vi "VSCode-dummy.vi"(11 "Enter your IP address":string="10.0.0.161") -> (0 "output cluster":errorcluster, 3 "standard output":string="Linux ev3dev 4.14.117-ev3dev-2.3.4-ev3 #1 PREEMPT Thu May 9 15:13:01 CDT 2019 armv5tejl\n             _____     _\n   _____   _|___ /  __| | _____   __\n  / _ \\ \\ / / |_ \\ / _` |/ _ \\ \\ / /\n |  __/\\ V / ___) | (_| |  __/\\ V /\n  \\___| \\_/ |____/ \\__,_|\\___| \\_/\n\nDebian stretch on LEGO MINDSTORMS EV3!\n")   [LabVIEW 2019]
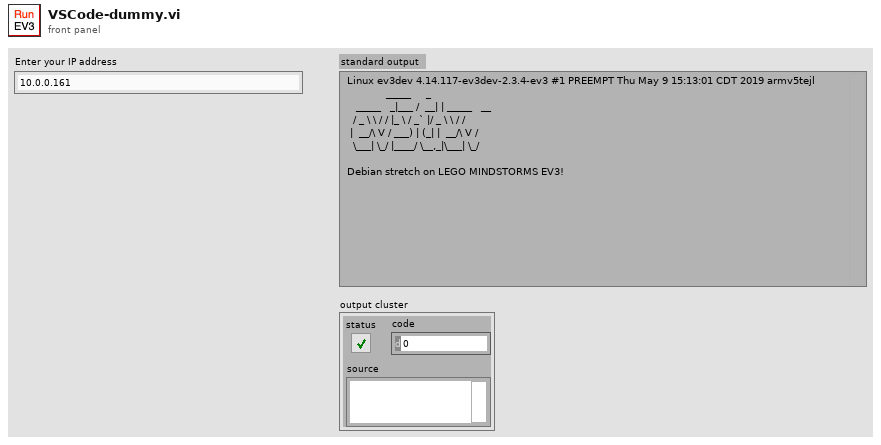
[diagram p1: front panel]
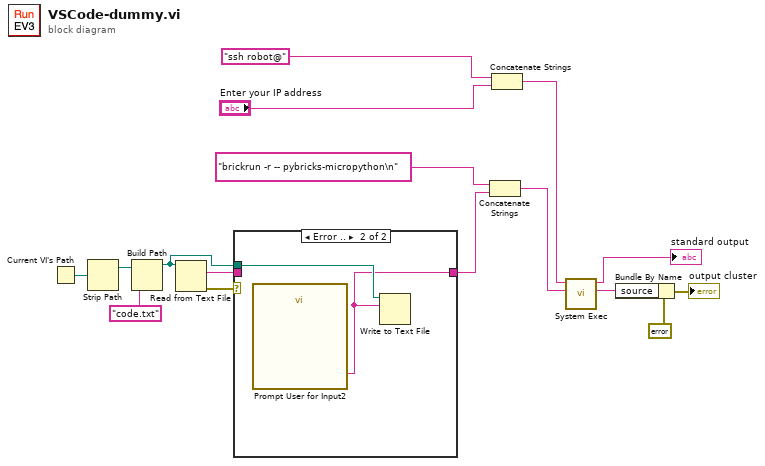
[diagram p0: block diagram]
diagram:
  n1 = Current VI's Path() -> (path=w15:path)
  n2 = Strip Path(path=w15) -> (stripped path=w14:path)  [unwired: 1 out]
  n3 = Build Path(base path=w14, name or relative path="code.txt") -> (appended path=w1:path)
  n4 = Read from Text File(file (use dialog)=w1) -> (text=w2:string, error out=w4:errorcluster)  [unwired: 3 in, 2 out]
  n5 = case shown="Error .." w4 {
    tunnel: w1 -> [_ w19]
    tunnel: [w17 w18] -> w3
    tunnel: w2 -> [w17 _]
    frame No Error {
    }
    frame Error {
      n6 = call "Prompt User for Input2"() -> ("code"=w18:string)  [unwired: 17 in, 2 out]
      n7 = Write to Text File(file (use dialog)=w19, text=w18) -> ()  [unwired: 2 in, 3 out]
    }
  }
  n8 = Concatenate Strings("brickrun -r -- pybricks-micropython\n" ("standard input"), w3) -> (w12:string)
  n9 = Concatenate Strings("ssh robot@" ("command line"), "Enter your IP address") -> (w11:string)
  n10 = call <vilib>:"System Exec.vi"("standard input"=w12, "command line"=w11) -> ("standard error"=w13:string, "standard output"=→"standard output":string)  [unwired: 6 in, 2 out]
  n11 = Bundle By Name(cluster=errorcluster {"status"=FALSE, "code"=0, "source"=""} ("error constant"), "source"=w13) -> (→"output cluster":errorcluster)
